vi "Charger_IPG VBAT Status.vi"(8 "error in":errorcluster, 10 "Charger Inputs":T1 {"setpoint" min=0.0 max=20000.0 step=100.0; "position" min=0 max=5 step=1}, 11 "MICS Dongle Address":refnum<visa-resource-name>="COM5") -> (0 "error out":errorcluster, 2 "VBAT":dbl=nan, 3 "ADC Counts":dbl=nan)   [LabVIEW 2020]
uses:
  Charger Test Set/Charger_Input Control.ctl
  Telemetry/Typedef Command List.ctl
panel:
  # "Get Telemetry from IPG"
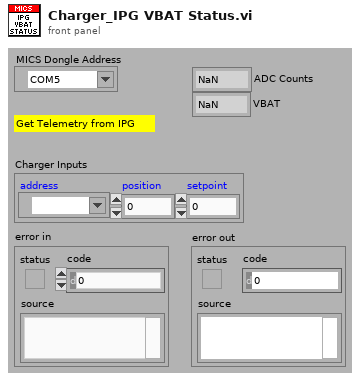
[diagram p1: front panel]
types:
  T1 = typedef "Charger_Input Control.ctl" = cluster{"address":refnum<visa-resource-name>, "position":i32, "setpoint":dbl}
  T2 = typedef "Typedef Command List.ctl" = enum16{"Get xPG Status", "xPG Stimulation", "Select Program", "Increment Program Amplitude", "Decrement Program Amplitude", "Get PoP Constants", "Get PPC Constants", "Get Program Names", "Set Pulse Amplitude", "Increment Pulse Amplitude", "Decrement Pulse Amplitude", "Get Pulse Widths", "Set Pulse Widths", "Increment Pulse Width", "Decrement Pulse Width", "Get Program Frequency", "Set Program Frequency", "Increment Program Frequency", "Decrement Program Frequency", "Inject Event", "Charging Control", "Get xPG Identity", "Set xPG Identity", "Restore Program Defaults", "Get Program Definition", "Set Program Definition", "Get Program Constants", "Set Program Constants", "Get Configurable Device Parameters", "Set Configurable Device Parameters", "Get Pulse Constants", "Set Pulse Constants", "Get Lead Limits", "Set Lead Limits", "Get Channel Calibrations", "Set Channel Calibrations", "<reserved 2>", "<reserved 3>", "<reserved 4>", "<reserved 5>", "<reserved 6>", "<reserved 7>", "Get Stim Asic HV Calibrations", "Set Stim Asic HV Calibrations", "<reserved 8>", "<reserved 9>", "Get CP Data", "Set CP Data", "Clear Log", "Read Log", "Append Log", "Get Patient Program Runtime", "Set Patient Program Runtime", "Impedance Measurement", "Enter Storage Mode", "Echo Short", "Echo Long", "Get General Calibration", "Set General Calibration", "Get Trim List", "Set Trim List", "Get Counter", "Set Counter", "Get Test Stimulation", "Set Test Stimulation", "Get Titration Stimulation", "Set Titration Stimulation", "Get Ramp Time", "Set Ramp Time", "Get VBAT", "Set Software Description Block", "Get Software Description Block", "Write Memory", "Read Memory", "Reset xPG", "Erase Flash Block", "Write Vectors", "Read Vectors", "Diagnostic Data", "Set Background Impedance", "Get Background Impedence ", "Set Test Waveform", "Calibrate Channel", "Get Log Range", "Reserved 0x55", "Reserved 0x56", "MICS Options", "Pair PPC", "Pair POP", "Stop Bootloader", "Tune MICS", "MICS Diagnostics", "Undefined"}
  T3 = cluster{"Command":T2, "Function":enum16{"Open Session", "Close Session", "Downlink Only", "Uplink Only", "Transceive (DN -> UP)"}, "MICS_ID":u32, "EXID":u32, "Use Local":bool, "Transceive Delay mS":dbl, "CP_DATA IN":u8[], "Parameters":string}
  T4 = enum16{"Open Session", "Close Session", "Downlink Only", "Uplink Only", "Transceive (DN -> UP)"}
  T5 = cluster{"Response Token":string, "Response Code":string, "bChecksum Valid":bool, "tChecksum Valid":bool, "CP_DATA OUT":u8[], "Data":string}
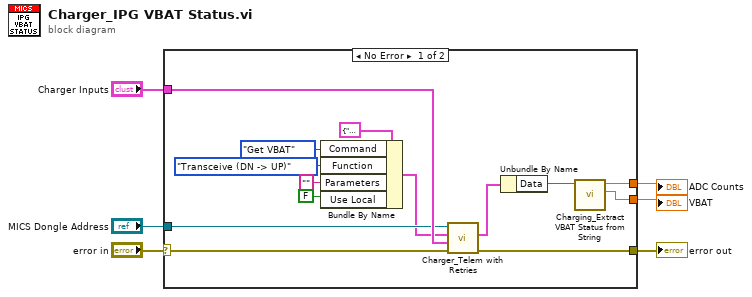
[diagram p0: block diagram]
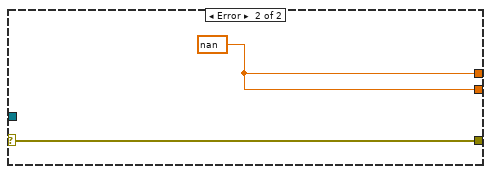
[diagram p2: hidden frame]
diagram:
  n1 = case shown="No Error" "error in" {
    selector: "error in" -> [w13 w22]
    tunnel: [w10 w22] -> w6
    tunnel: "MICS Dongle Address" -> [w11 _]
    tunnel: [w15 w21] -> w3
    tunnel: [w14 w21] -> w2
    tunnel: "Charger Inputs" -> [w12 _]
    frame No Error {
      n2 = Bundle By Name(cluster=T3 {"Command"=enum."Get xPG Status", "Function"=enum."Close Session", "MICS_ID"=0, "EXID"=16773121, "Use Local"=FALSE, "Transceive Delay mS"=100.0, "CP_DATA IN"=[], "Parameters"=""} ("Input"), "Command"=Typedef_Command_List."Get VBAT", "Function"=T4."Transceive (DN -> UP)", "Parameters"="", "Use Local"=FALSE) -> (w8:T3)
      n3 = call "Charger_Telem with Retries.vi"("error in"=w13, "Charger Inputs"=w12, "MICS Input"=w8, "MICS Dongle Address"=w11) -> ("error out"=w10:errorcluster, "Output"=w7:T5)  [unwired: 6 in]
      n4 = Unbundle By Name(w7) -> ("Data"=w16:string)
      n5 = call "Charging_Extract VBAT Status from String.vi"("Get VBAT String"=w16) -> ("VBAT (volts)"=w14:dbl, "ADC Counts"=w15:dbl)  [unwired: 9 in]
    }
    frame Error {
      w21 = nan ("VBAT (volts)")
    }
  }
  "error out" <- w6
  "ADC Counts" <- w3
  "VBAT" <- w2
